vi "getIgnoreMaxValue.vi"(8 "error in (no error)":errorcluster, 11 "ACNET Device in":refnum<class "ACNET Device.lvclass">) -> (0 "error out":errorcluster, 2 "ignoreMaxValue":bool, 3 "ACNET Device out":refnum<class "ACNET Device.lvclass">)   [LabVIEW 2013, in "ACNET Monitor.lvlib" / "ACNET Device.lvclass"]
uses:
  ACNET Device.lvclass
  ACNET Device.lvclass/ACNET Device.ctl
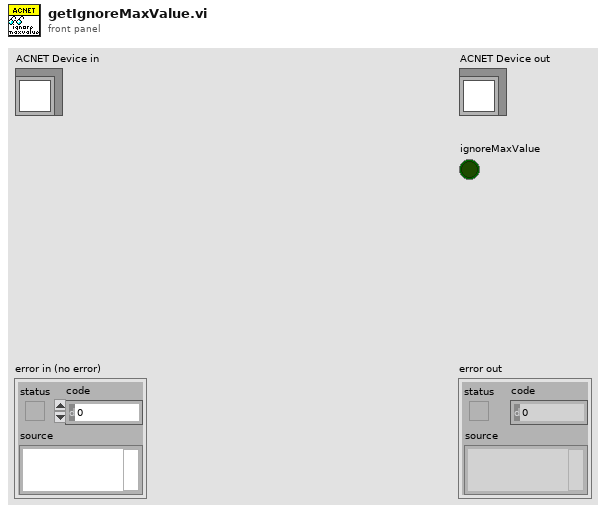
[diagram p1: front panel]
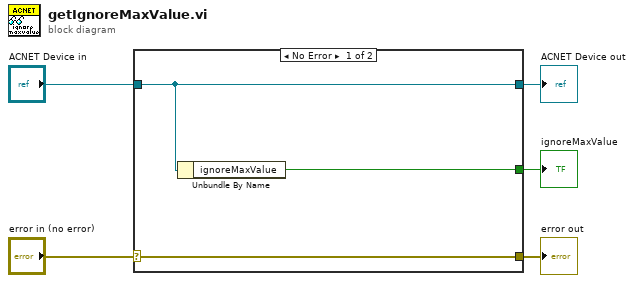
[diagram p0: block diagram]
diagram:
  n1 = case shown="No Error" "error in (no error)" {
    selector: "error in (no error)" -> [w8 w9]
    tunnel: [w8 w9] -> w4
    tunnel: [w7 w10] -> w2
    tunnel: "ACNET Device in" -> [w7 w10]
    tunnel: [w6 _] -> w1
    frame No Error {
      n2 = Unbundle By Name(w7) -> ("ignoreMaxValue"=w6:bool)
    }
    frame Error {
    }
  }
  "error out" <- w4
  "ACNET Device out" <- w2
  "ignoreMaxValue" <- w1
